vi "Valid Test Verification.vi"(0 "Parameters In":string[][](array[string]), 5 "Controller?":bool=TRUE, 7 "Flow":i32, 9 "Maxes":dbl[](array[numeric]), 11 "Mins":dbl[](array[numeric])) -> (4 "Parameters Out":string[][](array[string]), 6 "Valid?":bool, 8 "TimeValid?":bool, 10 "ProfileValid?":bool, 15 "NoCoerces":bool)   [LabVIEW 2013]
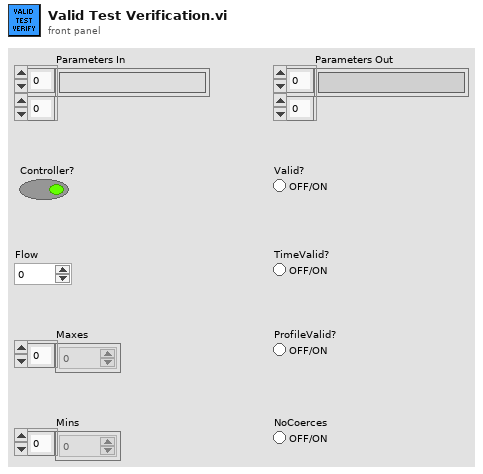
[diagram p1: front panel]
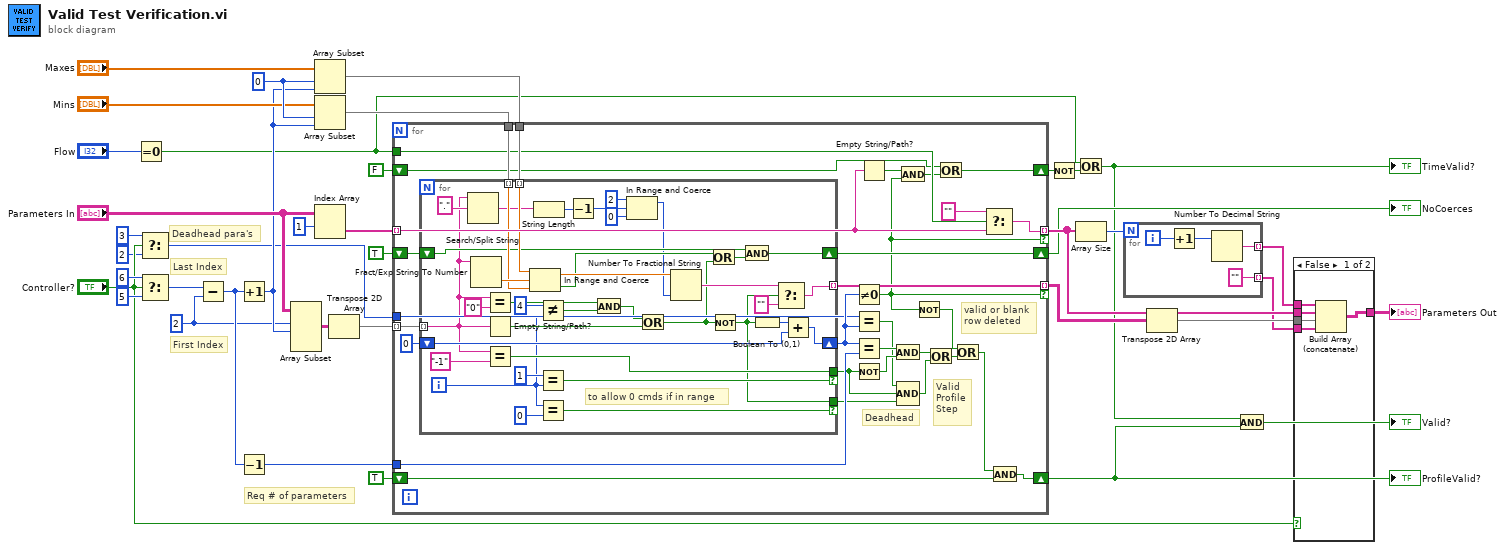
[diagram p0: block diagram]
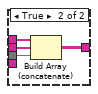
[diagram p2: hidden frame]
diagram:
  w9 = 2 ("y")
  w34 = 0 ("index")
  # "Req # of parameters"
  # "Deadhead para's"
  # "First Index"
  # "Last Index"
  n1 = Equal To 0?(x="Flow") -> (x = 0?=w10:bool)
  n2 = Select(t=3, s="Controller?", f=2) -> (s? t:f=w1:i32)
  n3 = Select(t=6, s="Controller?", f=5) -> (s? t:f=w37:i32)
  n4 = Subtract(x=w37, y=w9) -> (x-y=w36:i32)
  n5 = Increment(x=w36) -> (x+1=w16:i32)
  n6 = Decrement(x=w36) -> (x-1=w35:i32)
  n7 = Array Subset(array="Parameters In", index (row)=w9, length (row)=w16) -> (w27:string[][])  [unwired: 2 in]
  n8 = Array Subset(array="Maxes", index=w34, length=w16) -> (w31:dbl[])
  n9 = Array Subset(array="Mins", index=w34, length=w16) -> (w30:dbl[])
  n10 = Index Array(array="Parameters In", index (row)=1) -> (element=w25:string[])  [unwired: 1 in]
  n11 = Transpose 2D Array(2D array=w27) -> (transposed array=w26:string[][])
  n12 = for {
    tunnel: w26 -> [w69] mode=indexing
    tunnel: w35 -> [w68]
    tunnel: [w63] -> w21 mode=indexing if=w43
    tunnel: w31 -> [w67]
    tunnel: w30 -> [w66]
    shift-right: [w64] -> w7
    shift-left: TRUE -> [w65]
    tunnel: [w62] -> w22 mode=indexing if=w43
    tunnel: w25 -> [w55] mode=indexing
    tunnel: w10 -> [w61]
    shift-right: [w59] -> w8
    shift-left: TRUE -> [w58]
    shift-right: [w54] -> w12
    shift-left: FALSE -> [w41]
    tunnel: w1 -> [w40]
    # "valid or blank\nrow deleted"
    # "Valid\nProfile\nStep"
    # "Deadhead"
    n13 = for {
      tunnel: w69 -> [w78] mode=indexing
      shift-right: [w105] -> w49
      shift-left: i16 0 -> [w106]
      tunnel: [w103] -> w53 if=w101
      tunnel: [w91] -> w63 mode=indexing
      tunnel: w67 -> [w98] mode=indexing
      tunnel: w66 -> [w97] mode=indexing
      shift-right: [w95] -> w64
      shift-left: w65 -> [w96]
      tunnel: [w76] -> w57 if=w77
      i -> [w72]
      # "to allow 0 cmds if in range"
      n14 = Search/Split String(string=w78, search string/char (-)="." ("regular expression")) -> (match + rest of string=w88:string)  [unwired: 1 in, 2 out]
      n15 = Fract/Exp String To Number(string=w78) -> (number=w100:dbl)  [unwired: 3 in, 1 out]
      n16 = Equal?(x=w78, y="0") -> (x = y?=w75:bool)
      n17 = Empty String/Path?(string/path=w78) -> (empty?=w81:bool)
      n18 = Equal?(x=w78, y="-1") -> (x = y?=w103:bool)
      n19 = In Range and Coerce(upper limit=w98, x=w100, lower limit=w97) -> (coerced(x)=w99:dbl, In Range?=w94:bool)
      n20 = String Length(string=w88) -> (length=w87:i32)
      n21 = Not Equal?(x=4, y=w72) -> (x != y?=w73:bool)
      n22 = Equal?(x=1, y=w72) -> (x = y?=w101:bool)
      n23 = Equal?(x=w72, y=0 ("x")) -> (x = y?=w77:bool)
      n24 = Decrement(x=w87) -> (x-1=w86:i32)
      n25 = And(x=w75, y=w73) -> (x .and. y?=w74:bool)
      n26 = In Range and Coerce(upper limit=2, x=w86, lower limit=0) -> (coerced(x)=w85:i32)  [unwired: 1 out]
      n27 = Or(x=w74, y=w81) -> (x .or. y?=w80:bool)
      n28 = Number To Fractional String(number=w99, precision (6)=w85) -> (F-format string=w92:string)  [unwired: 2 in]
      n29 = Or(x=w94, y=w80) -> (x .or. y?=w93:bool)
      n30 = Not(x=w80) -> (.not. x?=w76:bool)
      n31 = And(x=w96, y=w93) -> (x .and. y?=w95:bool)
      n32 = Boolean To (0,1)(Boolean=w76) -> (0, 1=w107:i16)
      n33 = Select(t=w92, s=w76, f="") -> (s? t:f=w91:string)
      n34 = Add(x=w107, y=w106) -> (x+y=w105:i16)
    }
    n35 = Not Equal To 0?(x=w49) -> (x != 0?=w43:bool)
    n36 = Equal?(x=w40, y=w49) -> (x = y?=w48:bool)
    n37 = Equal?(x=w49, y=w68) -> (x = y?=w51:bool)
    n38 = Not(x=w53) -> (.not. x?=w52:bool)
    n39 = Empty String/Path?(string/path=w55) -> (empty?=w44:bool)
    n40 = And(x=w51, y=w52) -> (x .and. y?=w50:bool)
    n41 = Compound Arithmetic op=AND(w48, w53, w57) -> (w56:bool)
    n42 = And(x=w44, y=w43) -> (x .and. y?=w42:bool)
    n43 = Not(x=w43) -> (.not. x?=w47:bool)
    n44 = Or(x=w50, y=w56) -> (x .or. y?=w46:bool)
    n45 = Or(x=w41, y=w42) -> (x .or. y?=w54:bool)
    n46 = Or(x=w47, y=w46) -> (x .or. y?=w45:bool)
    n47 = Select(t="", s=w61, f=w55) -> (s? t:f=w62:string)
    n48 = And(x=w45, y=w58) -> (x .and. y?=w59:bool)
  }
  "NoCoerces" <- w7
  "ProfileValid?" <- w8
  n49 = Not(x=w12) -> (.not. x?=w11:bool)
  n50 = Or(x=w10, y=w11) -> (x .or. y?=w6:bool)
  "TimeValid?" <- w6
  n51 = Array Size(array=w22) -> (size(s)=w24:i32)
  n52 = for {
    N: w24 -> [_]
    tunnel: [w109] -> w23 mode=indexing
    tunnel: ["" ("t")] -> w19 mode=indexing
    i -> [w111]
    n53 = Increment(x=w111) -> (x+1=w110:i32)
    n54 = Number To Decimal String(number=w110) -> (decimal integer string=w109:string)  [unwired: 1 in]
  }
  n55 = Transpose 2D Array(2D array=w21) -> (transposed array=w20:string[][])
  n56 = And(x=w6, y=w8) -> (x .and. y?=→"Valid?":bool)
  n57 = case shown="False" "Controller?" {
    tunnel: w23 -> [w116 w120]
    tunnel: w22 -> [w115 w119]
    tunnel: w20 -> [w114 w118]
    tunnel: w19 -> [w113 _]
    tunnel: [w112 w117] -> w18
    frame False {
      n58 = Build Array (concatenate)(w116, w115, w114, w113) -> (w112:string[][])
    }
    frame True {
      n59 = Build Array (concatenate)(w120, w119, w118) -> (w117:string[][])
    }
  }
  "Parameters Out" <- w18
